vi "Wait to use camera.vi"(1 "error in":errorcluster) -> (0 "error out":errorcluster)   [LabVIEW 2016]
uses:
  camera globals.vi
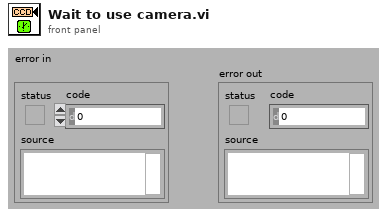
[diagram p1: front panel]
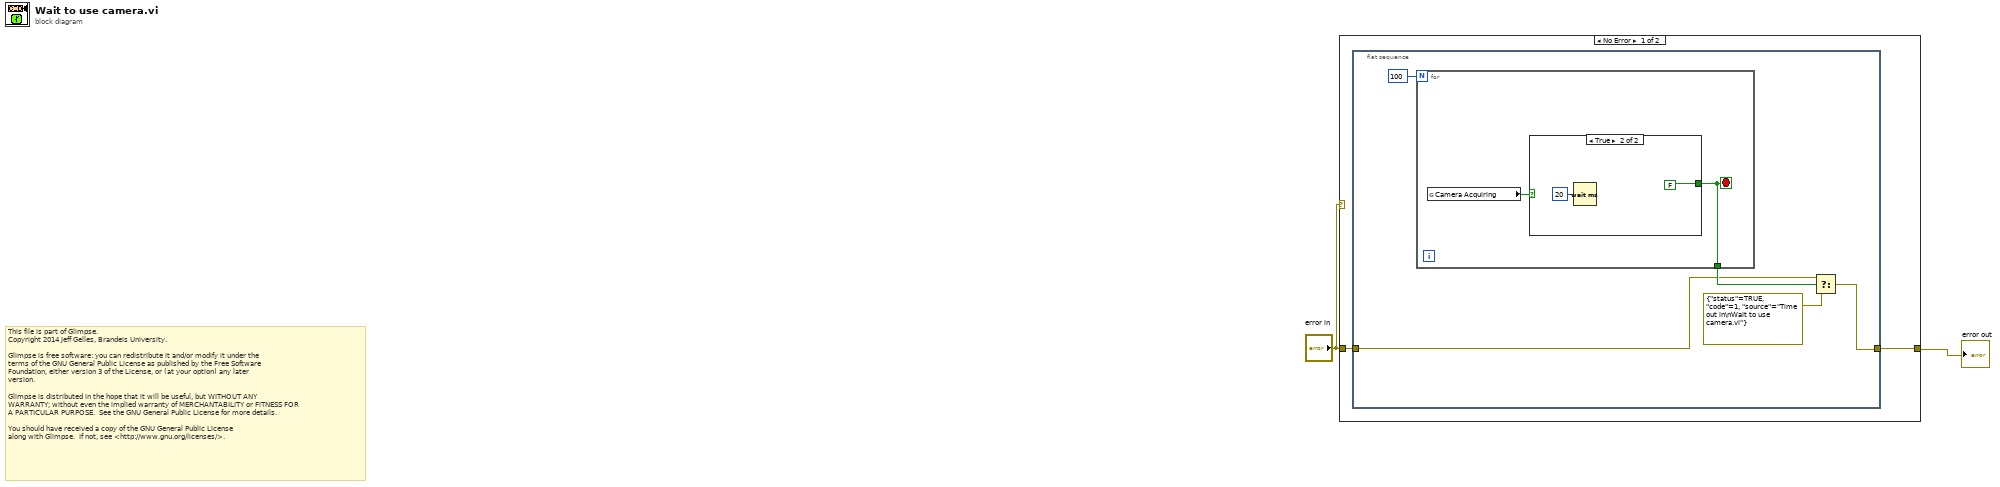
[diagram p0: block diagram]
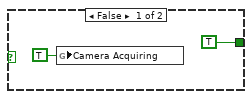
[diagram p2: hidden frame]
diagram:
  # "This file is part of Glimpse. \nCopyright 2014 Jeff Gelles, Brandeis University.    \n\nGlimpse is free software: you can redistribute it and/or modify it under the \nterms of the GNU General Public License as published by the Free Software \nFoundation, either version 3 of the License, or (at your option) any later \nversion.\n\nGlimpse is distributed in the hope that it will be useful, but WITHOUT ANY \nWARRANTY; without even the implied warranty of MERCHANTABILITY or FITNESS FOR \nA PARTICULAR PURPOSE.  See the GNU General Public License for more details.\n\nYou should have received a copy of the GNU General Public License\nalong with Glimpse.  If not, see <http://www.gnu.org/licenses/>."
  n1 = case shown="No Error" "error in" {
    tunnel: [w4 w16] -> w2
    tunnel: "error in" -> [w3 w16]
    frame No Error {
      n2 = flat-sequence {
        tunnel: w3 -> [w6]
        tunnel: [w8] -> w4
        frame #0 {
          n3 = for {
            N: 100 ("Numeric") -> [_]
            tunnel: [w10] -> w7
            stop <- w10 stop-if-true
            n4 = global read "camera globals.vi" "Camera Acquiring"() -> (w11:bool)
            n5 = case shown="True" w11 {
              tunnel: [TRUE FALSE] -> w10
              frame False {
                n6 = global write "camera globals.vi" "Camera Acquiring"(TRUE ("Camera Acquiring")) -> ()
              }
              frame True {
                n7 = Wait (ms)(milliseconds to wait=u32 20) -> ()  [unwired: 1 out]
              }
            }
          }
          n8 = Select(t=w6, s=w7, f=errorcluster {"status"=TRUE, "code"=1, "source"="Time out in\nWait to use camera.vi"}) -> (s? t:f=w8:errorcluster)
        }
      }
    }
    frame Error {
    }
  }
  "error out" <- w2
